vi "Init.vi"(1 "Baud Rate 2":u32=9600, 2 "# Port":refnum<visa-resource-name>) -> (0 "VISA resource name out":refnum<visa-resource-name>)   [LabVIEW 2020]
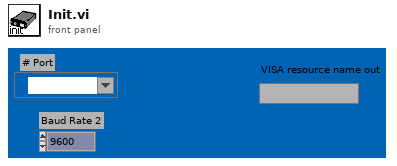
[diagram p1: front panel]
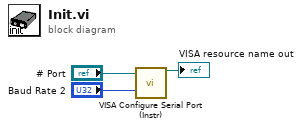
[diagram p0: block diagram]
diagram:
  n1 = call "VISA Configure Serial Port (Instr).vi"("VISA resource name"="# Port", "baud rate (9600)"="Baud Rate 2") -> ("VISA resource name out"=→"VISA resource name out":refnum<visa-resource-name>)  [unwired: 12 in, 1 out]
